vi "Save-Load Triggers Output Setup.vi"(6 "Which file? (User profile.ini)":T1=enum."Loaded User profile.ini", 8 "error in":errorcluster, 9 "Triggers output setup to save":T2=[{"Name"="Unused", "Output?"=FALSE, "Output terminal"="/PXI1Slot6/PFI0", "PXI backplane line"="/PXI1Slot6/PXI_Trig0", "Pulse width (us)"=20}, {"Name"="Line trigger", "Output?"=FALSE, "Output terminal"="/PXI1Slot6/PFI1", "PXI backplane line"="/PXI1Slot6/PXI_Trig1", "Pulse width (us)"=20}, {"Name"="Frame trigger / Trial trigger", "Output?"=FALSE, "Output terminal"="/PXI1Slot6/PFI2", "PXI backplane line"="/PXI1Slot6/PXI_Trig2", "Pulse width (us)"=20}, {"Name"="Cycle trigger", "Output?"=FALSE, "Output terminal"="/PXI1Slot6/PFI3", "PXI backplane line"="/PXI1Slot6/PXI_Trig3", "Pulse width (us)"=20}, {"Name"="Start of Experiment trigger", "Output?"=FALSE, "Output terminal"="/PXI1Slot6/PFI4", "PXI backplane line"="/PXI1Slot6/PXI_Trig4", "Pulse width (us)"=20}, {"Name"="Stimulus trigger", "Output?"=FALSE, "Output terminal"="/PXI1Slot6/PFI5", "PXI backplane line"="/PXI1Slot6/PXI_Trig5", "Pulse width (us)"=20}] {"Pulse width (us)" min=10 max=5000 step=1 format="%.0fµs"}, 11 "Function":T4=enum."Load from file") -> (0 "error out":errorcluster, 1 "Triggers output setup":T2=[{"Name"="", "Output?"=FALSE, "Output terminal"="/PXI1Slot6/PFI0", "PXI backplane line"="/PXI1Slot6/PXI_Trig0", "Pulse width (us)"=20}, {"Name"="", "Output?"=FALSE, "Output terminal"="/PXI1Slot6/PFI0", "PXI backplane line"="/PXI1Slot6/PXI_Trig0", "Pulse width (us)"=20}, {"Name"="", "Output?"=FALSE, "Output terminal"="/PXI1Slot6/PFI0", "PXI backplane line"="/PXI1Slot6/PXI_Trig0", "Pulse width (us)"=20}, {"Name"="", "Output?"=FALSE, "Output terminal"="/PXI1Slot6/PFI0", "PXI backplane line"="/PXI1Slot6/PXI_Trig0", "Pulse width (us)"=20}, {"Name"="", "Output?"=FALSE, "Output terminal"="/PXI1Slot6/PFI0", "PXI backplane line"="/PXI1Slot6/PXI_Trig0", "Pulse width (us)"=20}, {"Name"="", "Output?"=FALSE, "Output terminal"="/PXI1Slot6/PFI0", "PXI backplane line"="/PXI1Slot6/PXI_Trig0", "Pulse width (us)"=20}] {"Pulse width (us)" min=10 max=5000 step=1 format="%.0fµs"})   [LabVIEW 2013]
uses:
  Typedefs/Save-Load enum.ctl
  Peripherals Control/Triggers/Typedefs/Triggers output setup.ctl
  Peripherals Control/Triggers/Typedefs/Trigger setup element cluster.ctl
  Typedefs/Which path.ctl
  <vilib>/Utility/config.llb/NI_LVConfig.lvlib
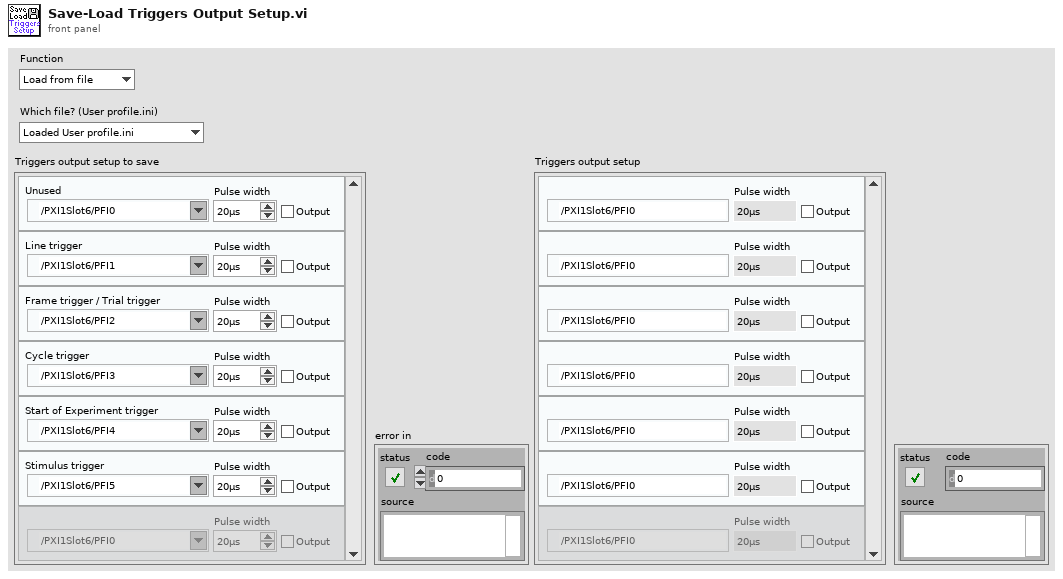
[diagram p1: front panel]
types:
  T1 = typedef "Which path.ctl" = enum16{"Configuration Files", "Calibration Files", "Images", "Setup.ini", "Loaded User profile.ini", "User's-Previous session.ini", "New user profile.ini", "Selected User profile.ini", "User profiles folder", "Power meter scaling.txt", "FOV Cal.ini"}
  T2 = typedef "Triggers output setup.ctl" = T3[]
  T3 = typedef "Trigger setup element cluster.ctl" = cluster{"Name":string, "Output?":bool, "Output terminal":tag, "PXI backplane line":tag, "Pulse width (us)":u16}
  T4 = typedef "Save-Load enum.ctl" = enum16{"Save to file", "Load from file", "Compare from file"}
  T5 = typedef "NI_LVConfig.lvlib/Config Data RefNum.ctl" = refnum<k1>
  T6 = typedef "Ini file interface (String).ctl" = cluster{"key":string, "Save?":bool, "Default":string}[]
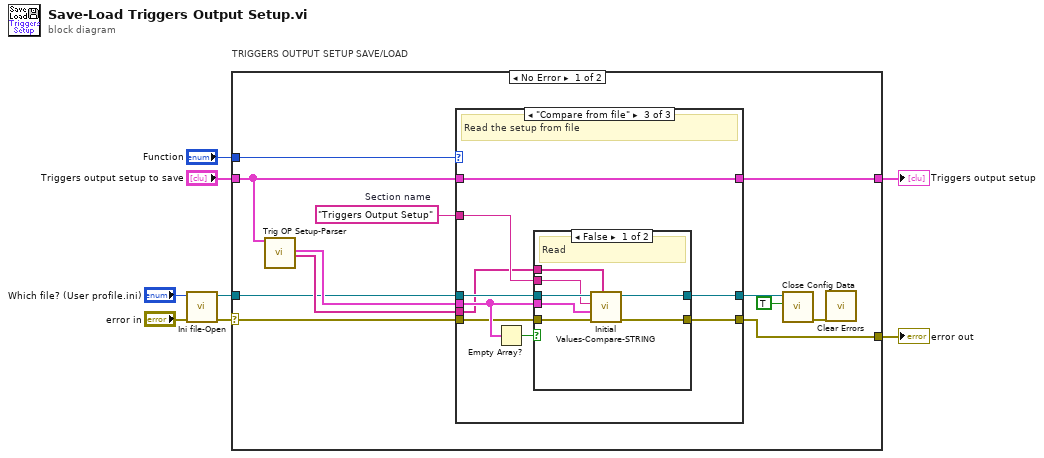
[diagram p0: block diagram]
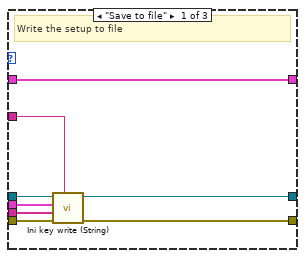
[diagram p2: hidden frame]
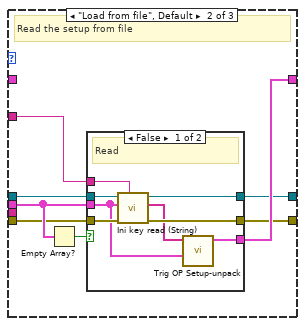
[diagram p3: hidden frame]
diagram:
  n1 = call "Ini file-Open.vi"("Error In"="error in", "Which file?"="Which file? (User profile.ini)") -> ("error out"=w7:errorcluster, "User profile ini file ref"=w5:T5)  [unwired: 6 in, 2 out]
  n2 = case "TRIGGERS OUTPUT SETUP SAVE/LOAD" shown="No Error" w7 {
    selector: w7 -> [w11 w66]
    tunnel: [w9 w66] -> w4
    tunnel: "Triggers output setup to save" -> [w15 w65]
    tunnel: [w16 w65] -> w2
    tunnel: "Function" -> [w12 _]
    tunnel: w5 -> [w10 _]
    frame No Error {
      w20 = "Triggers Output Setup"  # Section name
      n3 = call "Trig OP Setup-Parser.vi"("Triggers output setup to save"=w15) -> ("Keys setup"=w14:T6, "Values.Strings"=w13:string[])  [unwired: 17 in]
      n4 = case shown="\"Compare from file\"" w12 {
        tunnel: [w23 w30 w50] -> w9
        tunnel: [w24 w29 w49] -> w18
        tunnel: w11 -> [w21 w33 w52]
        tunnel: w10 -> [w22 w32 w51]
        tunnel: w20 -> [w26 w34 w53]
        tunnel: w13 -> [w27 _ w47]
        tunnel: w14 -> [w28 w35 w54]
        tunnel: [w25 w31 w48] -> w16
        tunnel: w15 -> [w25 _ w48]
        frame "Save to file" {
          # "Write the setup to file"
          n5 = call "Ini key write (String).vi"("Section"=w26, "error in (no error)"=w21, "Values (String)"=w27, "Ini file interface"=w28, "Ini file refnum in"=w22) -> ("error out"=w23:errorcluster, "Ini file refnum out"=w24:T5)  [unwired: 5 in]
        }
        frame "Load from file", Default {
          # "Read the setup from file"
          n6 = Empty Array?(array=w35) -> (empty?=w36:bool)
          n7 = case shown="False" w36 {
            tunnel: [w42 w46] -> w29
            tunnel: [w41 w45] -> w30
            tunnel: w35 -> [w37 _]
            tunnel: w32 -> [w44 w46]
            tunnel: w33 -> [w40 w45]
            tunnel: w34 -> [w43 _]
            tunnel: [w39 _] -> w31
            frame False {
              # "Read"
              n8 = call "Ini key read (String).vi"("Section name"=w43, "error in (no error)"=w40, "Keys setup"=w37, "Ini file ref in"=w44) -> ("error out"=w41:errorcluster, "Value read/used"=w38:string[], "Ini file ref"=w42:T5)  [unwired: 5 in]
              n9 = call "Trig OP Setup-unpack.vi"("Keys setup"=w37, "Value read/used"=w38) -> ("Triggers output setup"=w39:T2)  [unwired: 9 in]
            }
            frame True {
              # "Empty setup"
            }
          }
        }
        frame "Compare from file" {
          # "Read the setup from file"
          n10 = Empty Array?(array=w54) -> (empty?=w55:bool)
          n11 = case shown="False" w55 {
            tunnel: [w61 w64] -> w49
            tunnel: [w56 w63] -> w50
            tunnel: w54 -> [w59 _]
            tunnel: w51 -> [w62 w64]
            tunnel: w52 -> [w57 w63]
            tunnel: w53 -> [w60 _]
            tunnel: w47 -> [w58 _]
            frame False {
              # "Read"
              n12 = call "Initial Values-Compare-STRING.vi"("Current values"=w58, "error in (no error)"=w57, "Keys Array"=w59, "Section name"=w60, "User profile ini file ref"=w62) -> ("error out"=w56:errorcluster, "User profile ini file ref"=w61:T5)  [unwired: 2 in, 3 out]
            }
            frame True {
              # "Empty setup"
            }
          }
        }
      }
      n13 = call <vilib>:"Close Config Data.vi"("write file if changed (T)"=TRUE ("write configuration file? (F)"), "refnum"=w18) -> ("error out"=w17:errorcluster)  [unwired: 8 in, 1 out]
      n14 = call <vilib>:"Clear Errors.vi"("error in (no error)"=w17) -> ()  [unwired: 6 in, 1 out]
    }
    frame Error {
    }
  }
  "error out" <- w4
  "Triggers output setup" <- w2
